vi "Read Control Channel.vi"(8 "error in (no error)":errorcluster, 11 "Output in":refnum<class "Output.lvclass">) -> (0 "error out":errorcluster, 2 "Control Channel":bool, 3 "Output out":refnum<class "Output.lvclass">)   [LabVIEW 2023, in "HAF.lvlib" / "Output.lvclass"]
uses:
  Output.lvclass
  Output.lvclass/Output.ctl
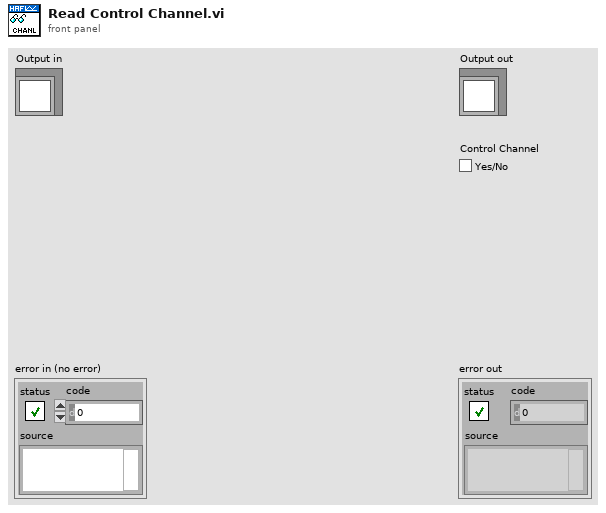
[diagram p1: front panel]
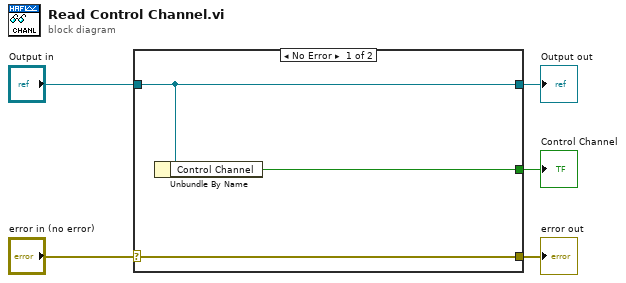
[diagram p0: block diagram]
diagram:
  n1 = case shown="No Error" "error in (no error)" {
    selector: "error in (no error)" -> [w8 w9]
    tunnel: [w8 w9] -> w4
    tunnel: [w7 w10] -> w2
    tunnel: "Output in" -> [w7 w10]
    tunnel: [w6 _] -> w1
    frame No Error {
      n2 = Unbundle By Name(w7) -> ("Control Channel"=w6:bool)
    }
    frame Error {
    }
  }
  "error out" <- w4
  "Output out" <- w2
  "Control Channel" <- w1
